vi "fgv_udp_remote-cmd.vi"(7 "cmd":enum16{"init", "read", "write", "close"}(ring), 8 "error in":errorcluster, 11 "data in":string) -> (0 "error out":errorcluster, 3 "data out":string)   [LabVIEW 2019]
panel:
  out "rd":string
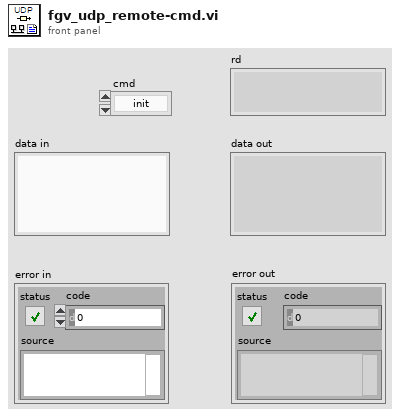
[diagram p1: front panel]
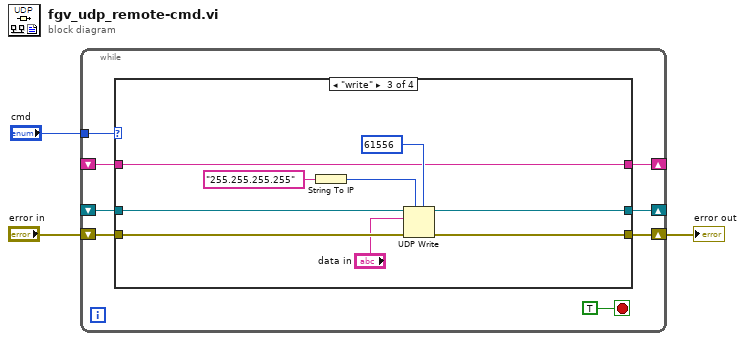
[diagram p0: block diagram]
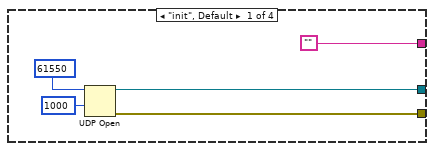
[diagram p2: hidden frame]
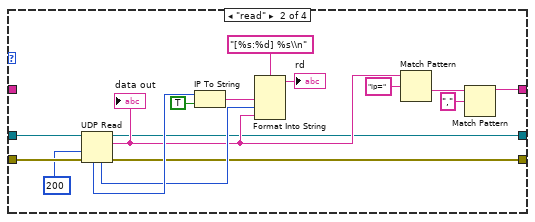
[diagram p3: hidden frame]
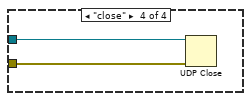
[diagram p4: hidden frame]
diagram:
  n1 = while {
    tunnel: "cmd" -> [w10]
    shift-right: [w9] -> _
    shift-left: _ -> [w6]
    shift-right: [w8] -> w1
    shift-left: "error in" -> [w7]
    shift-right: [w5] -> _
    shift-left: _ -> [w4]
    stop <- TRUE stop-if-true
    n2 = case shown="\"write\"" w10 {
      tunnel: [w16 w19 w39 _] -> w9
      tunnel: [w15 w18 w40 _] -> w8
      tunnel: w7 -> [_ w32 w41 w42]
      tunnel: w6 -> [_ w31 w38 w43]
      tunnel: ["" w17 w33 _] -> w5
      tunnel: w4 -> [_ _ w33 _]
      frame "init", Default {
        n3 = UDP Open(9:1000 ("타임아웃 ms (25000)"), 11:u16 61550 ("port")) -> (port=w16:refnum<k16>, 0:w15:errorcluster)  [unwired: 3 in, 1 out]
      }
      frame "read" {
        n4 = UDP Read(connection ID=w31, timeout ms (25000)=200, 8:w32) -> (data out=w23:string, error out=w18:errorcluster, 3:w19:refnum<k16>, 4:w25:u16, 6:w29:u32)  [unwired: 1 in]
        "data out" <- w23
        n5 = IP To String(1:TRUE ("점 표기? (거짓)"), 2:w29) -> (0:w27:string)
        n6 = Format Into String(format string="[%s:%d] %s\\n" ("포맷 문자열"), w27, w25, w23) -> (resulting string=→"rd":string)  [unwired: 2 in, 1 out]
        n7 = Match Pattern(string=w23, regular expression="ip=" ("정규식")) -> (after substring=w21:string)  [unwired: 1 in, 3 out]
        n8 = Match Pattern(string=w21, regular expression="," ("정규식")) -> (before substring=w17:string)  [unwired: 1 in, 3 out]
      }
      frame "write" {
        n9 = String To IP(1:"255.255.255.255" ("name")) -> (0:w34:u32)
        n10 = UDP Write(address=w34, port or service name=u16 61556, connection ID=w38, data in="data in", 8:w41) -> (error out=w40:errorcluster, 3:w39:refnum<k16>)  [unwired: 1 in]
      }
      frame "close" {
        n11 = UDP Close(connection ID=w43, 8:w42) -> ()  [unwired: 2 out]
      }
    }
  }
  "error out" <- w1
